vi "muti_channel_data_change.vi"(8 "Array - Numeric":dbl[](array[numeric]), 9 "?":T1(array[cluster]) {"Terminal Configuration" items=["default"=-1, "RSE"=10083, "NRSE"=10078, "Differential"=10106, "Pseudodifferential"=12529]}, 10 "data in":waveform(dbl)[](array[waveform])) -> (3 "data out":dbl[][](array[numeric]))   [LabVIEW 2024]
panel:
  out "empty channel":i32
  in  "element":waveform(dbl)
  out "data out":waveform(dbl)[](array[waveform])
  out "current channel":i32
  out "current begin channel":i32
  out "data size":i32
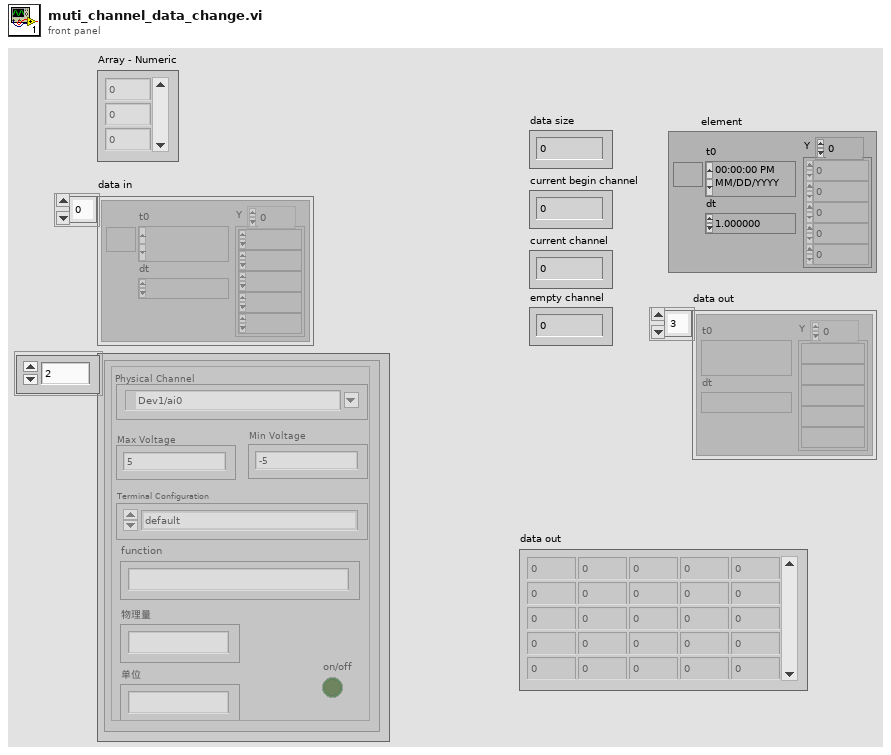
[diagram p1: front panel]
types:
  T1 = cluster{"Terminal Configuration":i32, "Min Voltage":dbl, "Physical Channel":tag, "Max Voltage":dbl, "function":string, "on/off":bool, "物理量":string, "单位":string}[]
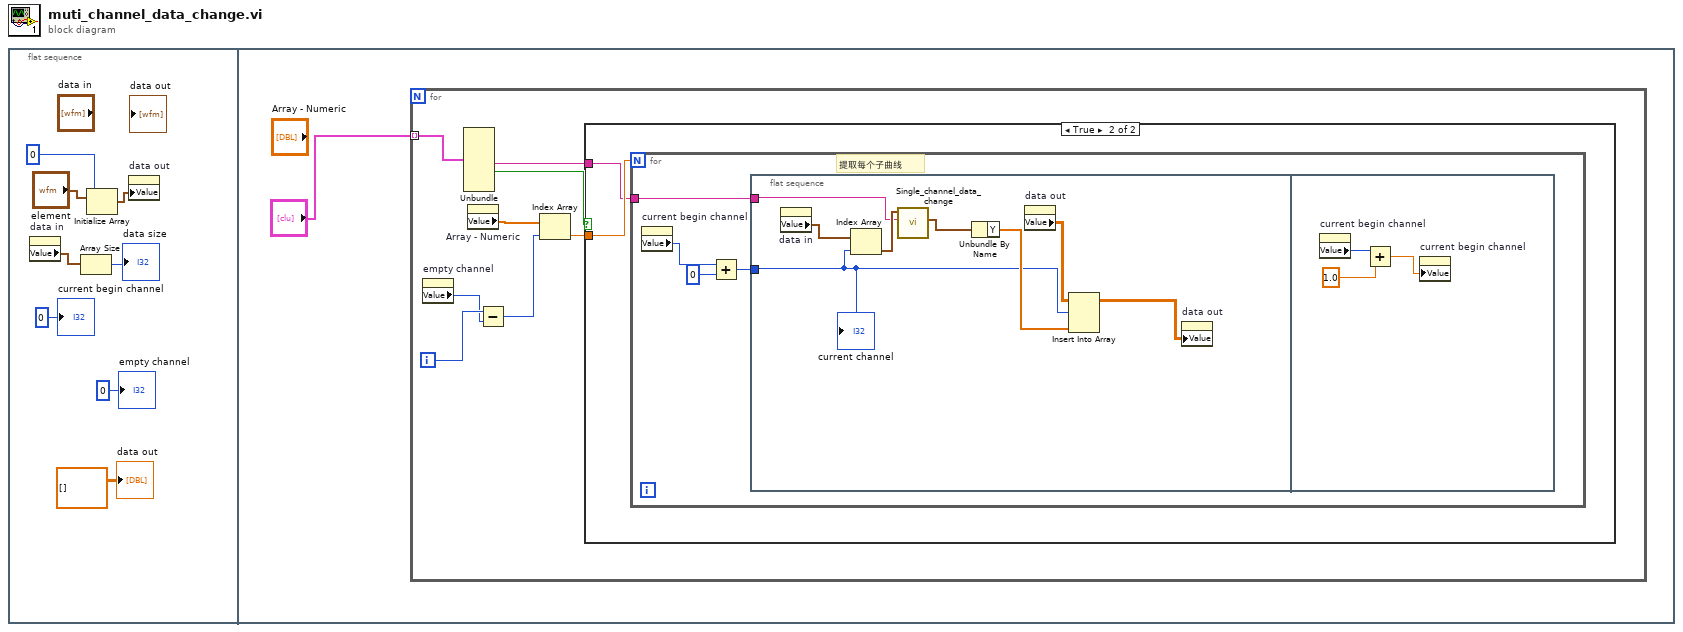
[diagram p0: block diagram]
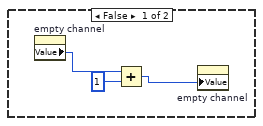
[diagram p2: hidden frame]
diagram:
  n1 = flat-sequence {
    frame #0 {
      n2 = property on="data in" class="Arr (strict)"() -> ("Value"=w8:waveform(dbl)[])  [unwired: 2 in, 2 out]
      n3 = Array Size(array=w8) -> (size(s)=→"data size":i32)
      n4 = Initialize Array("element", 0 ("dimension size")) -> (w3:waveform(dbl)[])
      n5 = property on="data out" class="Arr (strict)"("Value"=w3) -> ()  [unwired: 2 in, 2 out]
      "current begin channel" <- 0 ("current child channel")
      "empty channel" <- 0 ("empty channel")
      "data out" <- dbl[][] [] ("data out")
    }
    frame #1 {
      n6 = for {
        tunnel: "?" -> [w15] mode=indexing
        i -> [w12]
        n7 = property on="empty channel" class="DigNum (strict)"() -> ("Value"=w11:i32)  [unwired: 2 in, 2 out]
        n8 = Unbundle(w15) -> ("function"=w14:string, "on/off"=w13:bool)  [unwired: 6 out]
        n9 = property on="Array - Numeric" class="Arr (strict)"() -> ("Value"=w17:dbl[])  [unwired: 2 in, 2 out]
        n10 = Subtract(x=w12, y=w11) -> (x-y=w10:i32)
        n11 = Index Array(array=w17, index=w10) -> (element=w16:dbl)
        n12 = case shown="True" w13 {
          tunnel: w16 -> [_ w22]
          tunnel: w14 -> [_ w21]
          frame False {
            n13 = property on="empty channel" class="DigNum (strict)"() -> ("Value"=w20:i32)  [unwired: 2 in, 2 out]
            n14 = Add(x=w20, y=1) -> (x+y=w18:i32)
            n15 = property on="empty channel" class="DigNum (strict)"("Value"=w18) -> ()  [unwired: 2 in, 2 out]
          }
          frame True {
            n16 = for {
              N: w22 -> [_]
              tunnel: w21 -> [w24]
              # "提取每个子曲线"
              n17 = property on="current begin channel" class="DigNum (strict)"() -> ("Value"=w26:i32)  [unwired: 2 in, 2 out]
              n18 = Add(x=w26, y=0) -> (x+y=w25:i32)
              n19 = flat-sequence {
                tunnel: w25 -> [w28]
                tunnel: w24 -> [w32]
                frame #0 {
                  n20 = property on="data in" class="Arr (strict)"() -> ("Value"=w34:waveform(dbl)[])  [unwired: 2 in, 2 out]
                  n21 = Index Array(array=w34, index=w28) -> (element=w33:waveform(dbl))
                  n22 = call "Single_channel_data_change.vi"("String"=w32, "element in"=w33) -> ("element out"=w31:waveform(dbl))  [unwired: 9 in]
                  n23 = Unbundle By Name(w31) -> ("Y"=w29:dbl[])
                  n24 = property on="data out" class="Arr (strict)"() -> ("Value"=w30:dbl[][])  [unwired: 2 in, 2 out]
                  n25 = Insert Into Array(array=w30, index (row)=w28, new element=w29) -> (w27:dbl[][])  [unwired: 1 in]
                  n26 = property on="data out" class="Arr (strict)"("Value"=w27) -> ()  [unwired: 2 in, 2 out]
                  "current channel" <- w28
                }
                frame #1 {
                  n27 = property on="current begin channel" class="DigNum (strict)"() -> ("Value"=w36:i32)  [unwired: 2 in, 2 out]
                  n28 = Add(x=w36, y=1.0) -> (x+y=w35:dbl)
                  n29 = property on="current begin channel" class="DigNum (strict)"("Value"=w35) -> ()  [unwired: 2 in, 2 out]
                }
              }
            }
          }
        }
      }
    }
  }
